vi "DevControlPannel.vi"() -> ()   [LabVIEW 2017]
panel:
  in  "btnNewUserLib 3":bool
  in  "btnNewUserLib 2":bool
  in  "Experiments":i32(listbox)
  out "Current user path":path
  in  "btnExit":bool
  in  "btnLoadUserLib":bool
  in  "btnNewUserLib":bool
  in  "BtnNewExperiment":bool
  # "Select an experiment to open, or make the experiment into a template. (User new experiment create from templates)."
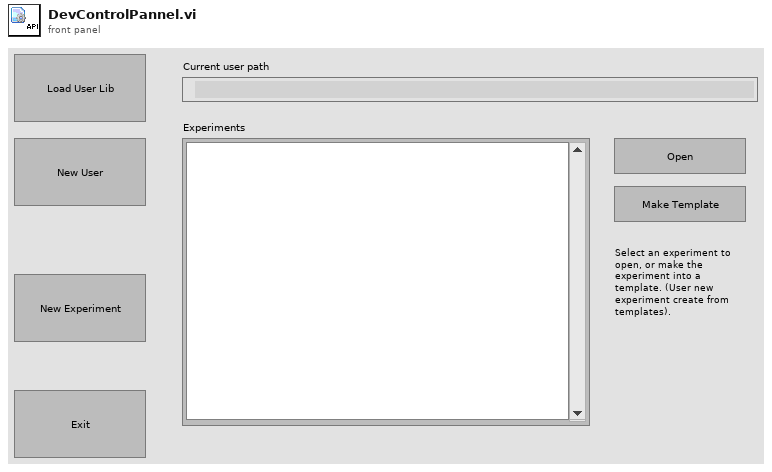
[diagram p1: front panel]
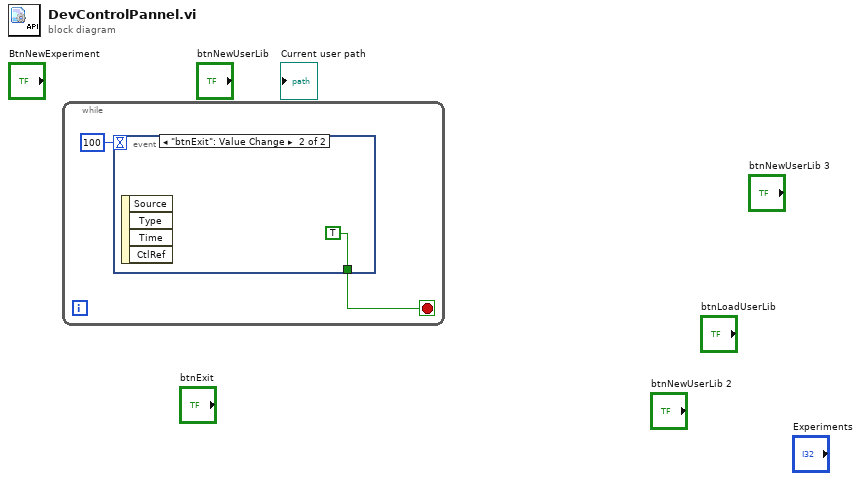
[diagram p0: block diagram]
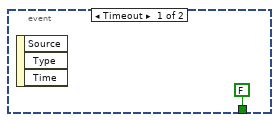
[diagram p2: hidden frame]
diagram:
  n1 = while {
    stop <- w1 stop-if-true
    n2 = event shown="[1] \"btnExit\": Value Change" {
      selector: _ -> [_ _]
      dyn-events: _ -> [_ _]
      timeout: 100 -> [_ _]
      tunnel: [FALSE TRUE] -> w1
      event Timeout {
        n3 = event-data() -> ()  [unwired: 1 in, 3 out]
      }
      event "btnExit": Value Change {
        n4 = event-data() -> ()  [unwired: 1 in, 4 out]
      }
    }
  }
